vi "readADC_ssxy.vi"(7 "x(0), y(0)":fxp<+/-,16,5>[](array[numeric]), 9 "z-err- ADC":refnum<k21>="Mod2/AI2", 10 "y - ADC":refnum<k21>="Mod2/AI1", 11 "x - ADC":refnum<k21>="Mod2/AI0") -> (2 "x_y_ze_z_k":fxp<+/-,17,6>[](array[numeric]))   [LabVIEW 2017]
uses:
  <vilib>/rvi/eio/common/nirviEmuTemplateMethod_errors.vi
  <vilib>/eio/EIONode/EIONode.xnode
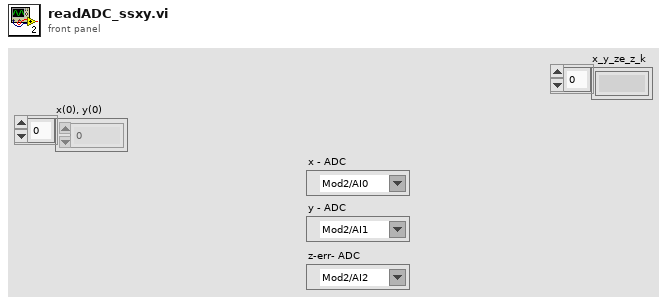
[diagram p1: front panel]
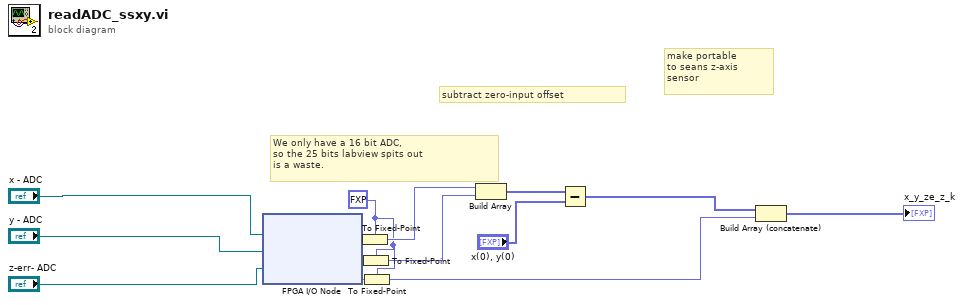
[diagram p0: block diagram]
diagram:
  w1 = fxp<+/-,16,5> 0.0 ("fixed-point type")
  # "We only have a 16 bit ADC,\nso the 25 bits labview spits out\nis a waste."
  # "make portable\nto seans z-axis\nsensor"
  # "subtract zero-input offset"
  n1 = xnode "FPGA I/O Node"("FPGA I/O In"="x - ADC", "FPGA I/O In"="y - ADC", "FPGA I/O In"="z-err- ADC") -> ("I/O Item"=w7:fxp<+/-,24,5>, "I/O Item"=w5:fxp<+/-,24,5>, "I/O Item"=w3:fxp<+/-,24,5>)  [unwired: 3 out]
  n2 = To Fixed-Point(fixed-point type=w1, number=w7) -> (fixed-point=w6:fxp<+/-,16,5>)
  n3 = To Fixed-Point(fixed-point type=w1, number=w5) -> (fixed-point=w4:fxp<+/-,16,5>)
  n4 = To Fixed-Point(fixed-point type=w1, number=w3) -> (fixed-point=w2:fxp<+/-,16,5>)
  n5 = Build Array(w6, w4) -> (w13:fxp<+/-,16,5>[])
  n6 = Subtract(x=w13, y="x(0), y(0)") -> (x-y=w11:fxp<+/-,17,6>[])
  n7 = Build Array (concatenate)(w11, w2) -> (→"x_y_ze_z_k":fxp<+/-,17,6>[])
